vi "Get Topic Rule Details.vi"(8 "error in (no error)":errorcluster, 10 "Rule Name":string, 11 "IoT Session in":refnum<class "IoT Session.lvclass">) -> (0 "error out":errorcluster, 2 "Topic Rule":T1, 3 "IoT Session out":refnum<class "IoT Session.lvclass">)   [LabVIEW 2015, in "NI_AWS_IoT.lvlib" / "IoT Session.lvclass"]
uses:
  IoT Session.lvclass
  Topic Rule.ctl
  CloudWatch Alarm.ctl
  CloudWatch Metric.ctl
  DynamoDB.ctl
  DynamoDBv2.ctl
  Elasticsearch.ctl
  Firehose.ctl
  Kinesis.ctl
  Lambda.ctl
  Republish.ctl
  S3.ctl
  SNS.ctl
  SQS.ctl
  Core/HTTP Request/Request Options.ctl
  Core/HTTP Request/Name Value Pair.ctl
  Core/HTTP Request/Region handling.ctl
  Core/HTTP Request/URL formatting.ctl
  Core/HTTP Request/HTTP Request.lvclass
  NI_AWS_IoT.lvlib
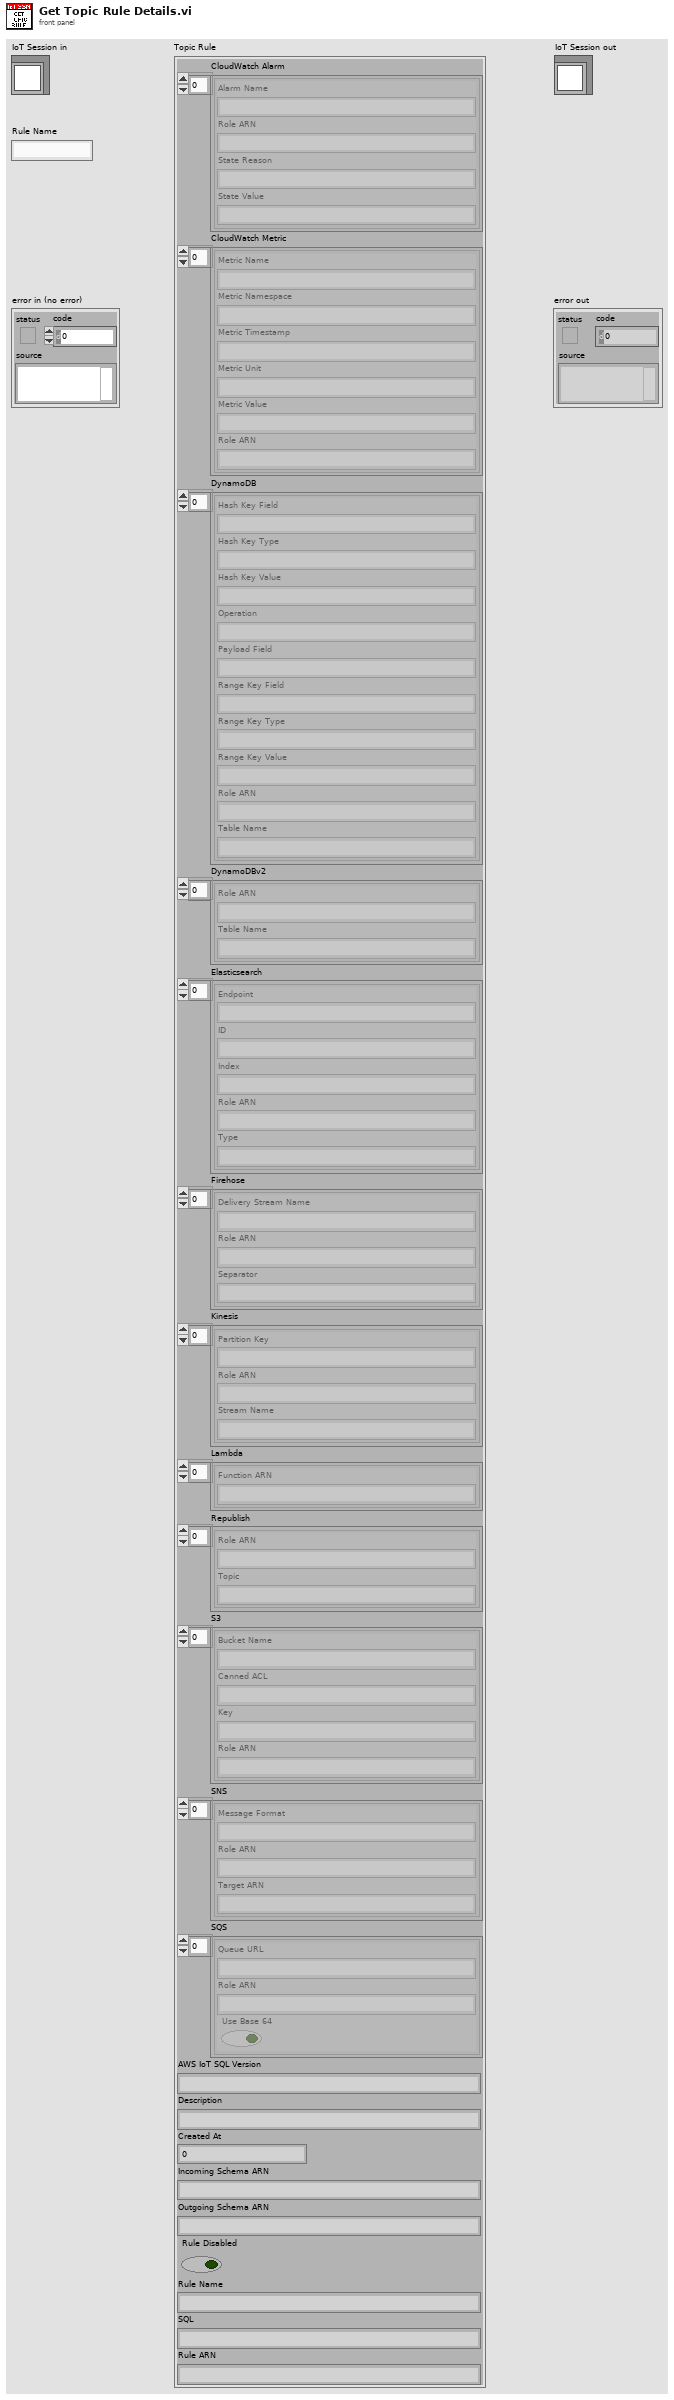
[diagram p1: front panel]
types:
  T1 = typedef "NI_AWS_IoT.lvlib/Topic Rule.ctl" = cluster{"CloudWatch Alarm":T2[], "CloudWatch Metric":T3[], "DynamoDB":T4[], "DynamoDBv2":T5[], "Elasticsearch":T6[], "Firehose":T7[], "Kinesis":T8[], "Lambda":T9[], "Republish":T10[], "S3":T11[], "SNS":T12[], "SQS":T13[], "AWS IoT SQL Version":string, "Description":string, "Created At":u64, "Incoming Schema ARN":string, "Outgoing Schema ARN":string, "Rule Disabled":bool, "Rule Name":string, "SQL":string, "Rule ARN":string}
  T2 = typedef "NI_AWS_IoT.lvlib/CloudWatch Alarm.ctl" = cluster{"Alarm Name":string, "Role ARN":string, "State Reason":string, "State Value":string}
  T3 = typedef "NI_AWS_IoT.lvlib/CloudWatch Metric.ctl" = cluster{"Metric Name":string, "Metric Namespace":string, "Metric Timestamp":string, "Metric Unit":string, "Metric Value":string, "Role ARN":string}
  T4 = typedef "NI_AWS_IoT.lvlib/DynamoDB.ctl" = cluster{"Hash Key Field":string, "Hash Key Type":string, "Hash Key Value":string, "Operation":string, "Payload Field":string, "Range Key Field":string, "Range Key Type":string, "Range Key Value":string, "Role ARN":string, "Table Name":string}
  T5 = typedef "NI_AWS_IoT.lvlib/DynamoDBv2.ctl" = cluster{"Role ARN":string, "Table Name":string}
  T6 = typedef "NI_AWS_IoT.lvlib/Elasticsearch.ctl" = cluster{"Endpoint":string, "ID":string, "Index":string, "Role ARN":string, "Type":string}
  T7 = typedef "NI_AWS_IoT.lvlib/Firehose.ctl" = cluster{"Delivery Stream Name":string, "Role ARN":string, "Separator":string}
  T8 = typedef "NI_AWS_IoT.lvlib/Kinesis.ctl" = cluster{"Partition Key":string, "Role ARN":string, "Stream Name":string}
  T9 = typedef "NI_AWS_IoT.lvlib/Lambda.ctl" = cluster{"Function ARN":string}
  T10 = typedef "NI_AWS_IoT.lvlib/Republish.ctl" = cluster{"Role ARN":string, "Topic":string}
  T11 = typedef "NI_AWS_IoT.lvlib/S3.ctl" = cluster{"Bucket Name":string, "Canned ACL":string, "Key":string, "Role ARN":string}
  T12 = typedef "NI_AWS_IoT.lvlib/SNS.ctl" = cluster{"Message Format":string, "Role ARN":string, "Target ARN":string}
  T13 = typedef "NI_AWS_IoT.lvlib/SQS.ctl" = cluster{"Queue URL":string, "Role ARN":string, "Use Base 64":bool}
  T14 = typedef "NI_AWS_Core.lvlib/HTTP Request.lvclass/Name Value Pair.ctl" = cluster{"name":string, "value":string}
  T15 = typedef "NI_AWS_Core.lvlib/HTTP Request.lvclass/Request Options.ctl" = cluster{"request headers":T14[], "request parameters":T14[], "request body":string, "region handling":T16, "URL formatting":T17}
  T16 = typedef "NI_AWS_Core.lvlib/HTTP Request.lvclass/Region handling.ctl" = enum16{"use region everywhere", "use region (authentication only)", "use region (URL only)", "ignore region everwhere"}
  T17 = typedef "NI_AWS_Core.lvlib/HTTP Request.lvclass/URL formatting.ctl" = enum16{"region-", "region."}
  T18 = typedef "NI_AWS_Core.lvlib/HTTP Request.lvclass/Response.ctl" = cluster{"Headers":string, "Body":string}
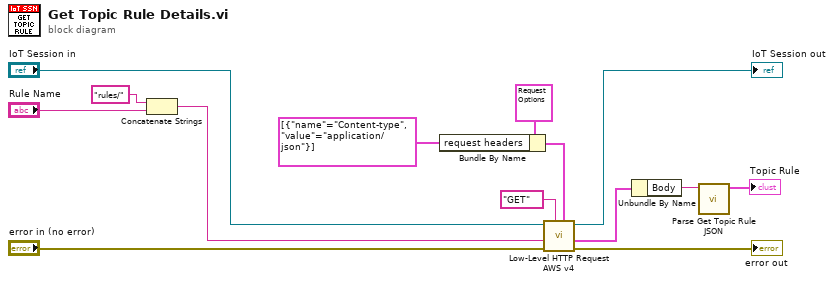
[diagram p0: block diagram]
diagram:
  n1 = Concatenate Strings("rules/" ("string"), "Rule Name") -> (w4:string)
  n2 = Bundle By Name(cluster=T15 {"request headers"=[], "request parameters"=[], "request body"="", "region handling"=enum."use region everywhere", "URL formatting"=enum."region."} ("Request Options"), "request headers"=T14[] [{"name"="Content-type", "value"="application/json"}]) -> (w12:T15)
  n3 = call "Low-Level HTTP Request AWS v4.vi"("Request Options"=w12, "HTTP-Verb"="GET", "error in (no error)"="error in (no error)", "URL Suffix"=w4, "AWS Core in"="IoT Session in") -> ("error out"=→"error out":errorcluster, "Response"=w3:T18, "AWS Core out"=→"IoT Session out":refnum<class "IoT Session.lvclass">)  [unwired: 3 in, 1 out]
  n4 = Unbundle By Name(w3) -> ("Body"=w2:string)
  n5 = call "Parse Get Topic Rule JSON.vi"("Body"=w2) -> ("Topic Rule"=→"Topic Rule":T1)  [unwired: 10 in]
